vi "SW_SG_coefficients.vi"(2 "1st order derivative? (F)":bool, 3 "Filter parameters":T1={"Filter type"=enum."Savitzky-Golay", "Length"=31, "Order"=3} {"Order" min=3 max=11 step=2; "Length" min=5 max=301 step=2}) -> (1 "SG filter coefficients":dbl[](array[numeric]))   [LabVIEW 2018, in "Tracker.lvlib"]
uses:
  Tracker.lvlib
  Controls/CTL_Filter_selector.ctl
  <vilib>/Analysis/NI_AALBase.lvlib
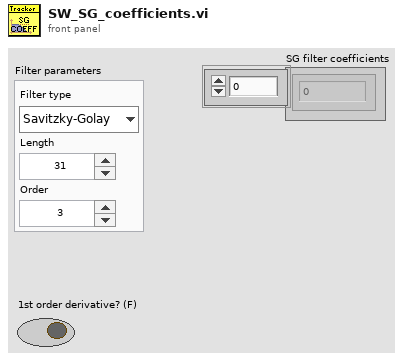
[diagram p1: front panel]
types:
  T1 = typedef "Tracker.lvlib/CTL_Filter_selector.ctl" = cluster{"Filter type":enum16{"None", "Savitzky-Golay"}, "Length":i32, "Order":i32}
  T2 = typedef "NI_Matrix.lvlib/RealMatrix.ctl" = dbl[][]
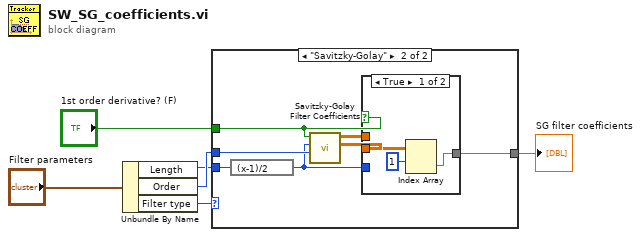
[diagram p0: block diagram]
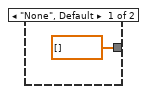
[diagram p2: hidden frame]
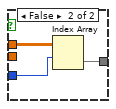
[diagram p3: hidden frame]
diagram:
  n1 = Unbundle By Name("Filter parameters") -> ("Length"=w5:i32, "Order"=w6:i32, "Filter type"=w3:enum16{"None", "Savitzky-Golay"})
  n2 = case shown="\"Savitzky-Golay\"" w3 {
    tunnel: w6 -> [_ w14]
    tunnel: w5 -> [_ w12]
    tunnel: [dbl[] [] ("Savitzky-Golay Filters") w10] -> w4
    tunnel: "1st order derivative? (F)" -> [_ w9]
    frame "None", Default {
    }
    frame "Savitzky-Golay" {
      n3 = expression code="(x-1)/2"(w12) -> (w11:i32)
      n4 = call <vilib>:"Savitzky-Golay Filter Coefficients.vi"("polynomial order"=w14, "side points"=w11, "compute differentiation filters?"=w9) -> ("Differentiation Filters"=w8:T2, "Savitzky-Golay Filters"=w13:T2)  [unwired: 6 in, 1 out]
      n5 = case shown="True" w9 {
        tunnel: w13 -> [_ w20]
        tunnel: w11 -> [_ w19]
        tunnel: [w17 w18] -> w10
        tunnel: w8 -> [w16 _]
        frame True {
          n6 = Index Array(array=w16, index (row)=1) -> (element=w17:dbl[])  [unwired: 1 in]
        }
        frame False {
          n7 = Index Array(array=w20, index (row)=w19) -> (element=w18:dbl[])  [unwired: 1 in]
        }
      }
    }
  }
  "SG filter coefficients" <- w4
